vi "Print Console.vi"() -> ()   [LabVIEW 2016]
doc: "This print queue console simulates the control of print job submissions and monitors the status of the print jobs being processed."
uses:
  Print Indicators.ctl
  Print Processing States.ctl
  <vilib>/Utility/error.llb/DialogType.ctl
panel:
  out "Print Indicators":T1={"Waiting"=TRUE, "Initializing"=FALSE, "Printing"=FALSE, "Job Number"=0}
  out "Queued Print Jobs":i32(slide) scale=0.0..25.0
  in  "Queue Event":bool
  in  "Stop":bool
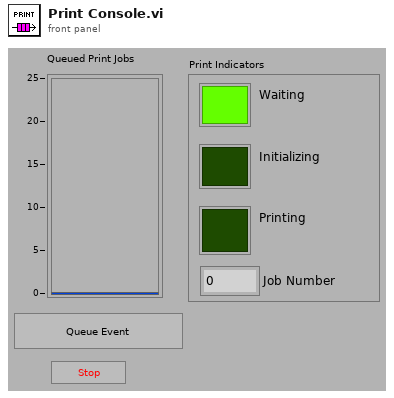
[diagram p1: front panel]
types:
  T1 = typedef "Print Indicators.ctl" = cluster{"Waiting":bool, "Initializing":bool, "Printing":bool, "Job Number":i32}
  T2 = typedef "DialogType.ctl" = u16
  T3 = typedef "Print Processing States.ctl" = enum16{"Wait", "Initialize Setup", "Setup", "Initialize Print", "Print", "Shutdown"}
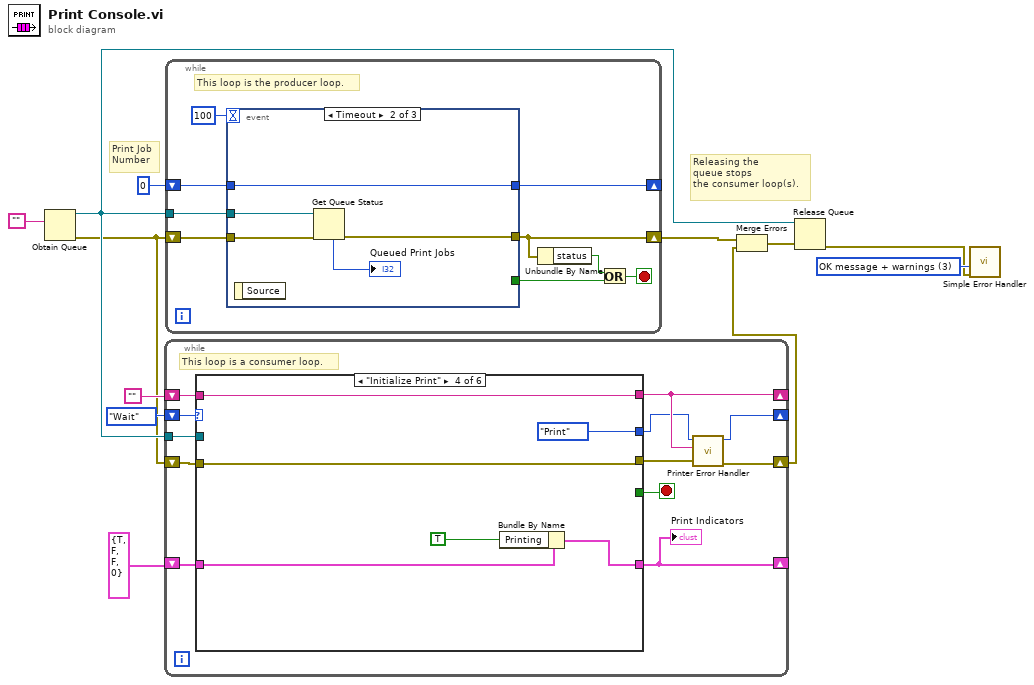
[diagram p0: block diagram]
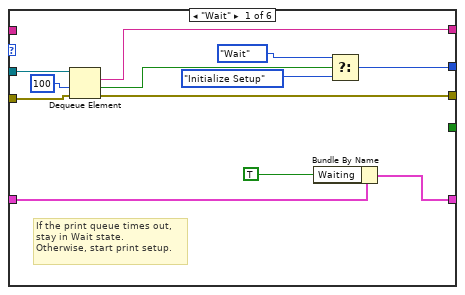
[diagram p2: hidden frame]
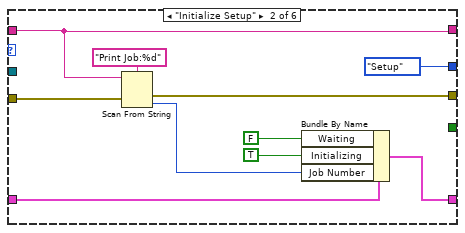
[diagram p3: hidden frame]
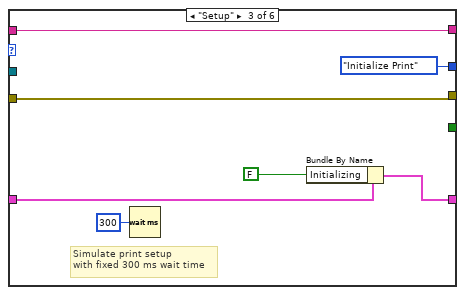
[diagram p4: hidden frame]
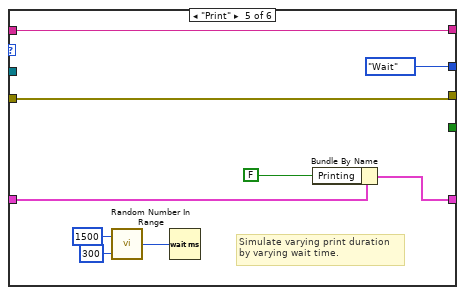
[diagram p5: hidden frame]
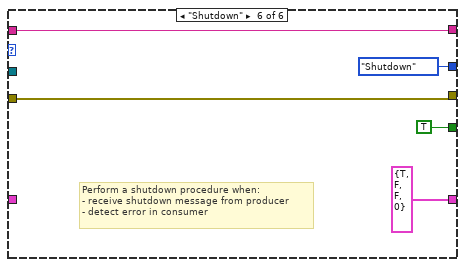
[diagram p6: hidden frame]
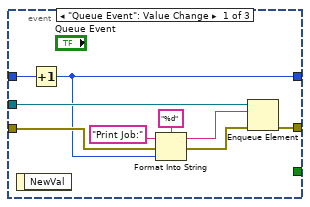
[diagram p7: hidden frame]
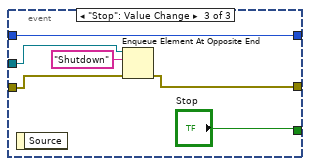
[diagram p8: hidden frame]
diagram:
  w5 = T2 3 items=["no dialog", "OK message", "continue or stop message", "OK message + warnings", "continue/stop + warnings"] ("type of dialog (OK msg:1)")
  # "Print Job\nNumber"
  # "Releasing the\nqueue stops\nthe consumer loop(s)."
  n1 = Obtain Queue(element data type="") -> (queue out=w11:refnum<queue>, error out=w6:errorcluster)  [unwired: 4 in, 1 out]
  n2 = while {
    tunnel: w11 -> [w24]
    shift-right: [w13] -> _
    shift-left: Print_Processing_States."Wait" ("Enum") -> [w23]
    shift-right: [w21] -> _
    shift-left: T1 {"Waiting"=TRUE, "Initializing"=FALSE, "Printing"=FALSE, "Job Number"=0} ("Print LEDs") -> [w22]
    shift-right: [w15] -> _
    shift-left: "" -> [w20]
    shift-right: [w16] -> w1
    shift-left: w6 -> [w19]
    stop <- w18 stop-if-true
    # "This loop is a consumer loop."
    n3 = case shown="\"Initialize Print\"" w23 {
      tunnel: w24 -> [w36 _ _ _ _ _]
      tunnel: [w35 w38 w47 w54 w60 w70] -> w17
      tunnel: w22 -> [w30 w45 w52 w58 w67 _]
      tunnel: [w29 w44 w51 w57 w66 T1 {"Waiting"=TRUE, "Initializing"=FALSE, "Printing"=FALSE, "Job Number"=0} ("Print LEDs")] -> w21
      tunnel: [w27 Print_Processing_States."Setup" ("Enum") Print_Processing_States."Initialize Print" ("Enum") Print_Processing_States."Print" ("Enum") Print_Processing_States."Wait" ("Enum") Print_Processing_States."Shutdown" ("Enum")] -> w14
      tunnel: [w26 w41 w48 w55 w61 w71] -> w15
      tunnel: w20 -> [_ w41 w48 w55 w61 w71]
      tunnel: w19 -> [w25 w37 w47 w54 w60 w70]
      tunnel: [_ _ _ _ _ TRUE] -> w18
      frame "Wait" {
        # "If the print queue times out, \nstay in Wait state.\nOtherwise, start print setup."
        n4 = Dequeue Element(queue=w36, timeout in ms (-1)=100, error in (no error)=w25) -> (element=w26:string, timed out?=w28:bool, error out=w35:errorcluster)  [unwired: 1 out]
        n5 = Bundle By Name(cluster=w30, "Waiting"=TRUE ("Waiting for\nnew job...")) -> (w29:T1)
        n6 = Select(t=Print_Processing_States."Wait" ("Enum"), s=w28, f=Print_Processing_States."Initialize Setup" ("Enum")) -> (s? t:f=w27:T3)
      }
      frame "Initialize Setup" {
        n7 = Scan From String(format string="Print Job:%d", input string=w41, error in=w37) -> (error out=w38:errorcluster, output 1=w39:i32)  [unwired: 2 in, 2 out]
        n8 = Bundle By Name(cluster=w45, "Waiting"=FALSE ("Waiting for\nnew job..."), "Initializing"=TRUE ("Waiting for\nnew job..."), "Job Number"=w39) -> (w44:T1)
      }
      frame "Setup" {
        # "Simulate print setup\nwith fixed 300 ms wait time"
        n9 = Wait (ms)(milliseconds to wait=u32 300) -> ()  [unwired: 1 out]
        n10 = Bundle By Name(cluster=w52, "Initializing"=FALSE ("Waiting for\nnew job...")) -> (w51:T1)
      }
      frame "Initialize Print" {
        n11 = Bundle By Name(cluster=w58, "Printing"=TRUE ("Waiting for\nnew job...")) -> (w57:T1)
      }
      frame "Print" {
        # "Simulate varying print duration\nby varying wait time."
        n12 = call "Random Number In Range.vi"("Lower Limit"=u32 300, "Upper Limit"=u32 1500) -> ("Random #"=w62:u32)
        n13 = Wait (ms)(milliseconds to wait=w62) -> ()  [unwired: 1 out]
        n14 = Bundle By Name(cluster=w67, "Printing"=FALSE ("Waiting for\nnew job...")) -> (w66:T1)
      }
      frame "Shutdown" {
        # "Perform a shutdown procedure when:\n- receive shutdown message from producer\n- detect error in consumer"
      }
    }
    "Print Indicators" <- w21
    n15 = call "Printer Error Handler.vi"("error in (no error)"=w17, "Queue Data"=w15, "State In"=w14) -> ("error out"=w16:errorcluster, "Next State"=w13:T3)  [unwired: 7 in]
  }
  n16 = while {
    tunnel: w11 -> [w82]
    shift-right: [w76] -> _
    shift-left: 0 -> [w77]
    shift-right: [w75] -> w4
    shift-left: w6 -> [w74]
    stop <- w80 stop-if-true
    # "This loop is the producer loop."
    n17 = event shown="[1] Timeout" {
      selector: _ -> [_ _ _]
      dyn-events: _ -> [_ _ _]
      timeout: 100 -> [_ _ _]
      tunnel: w82 -> [w91 w94 w97]
      tunnel: w74 -> [w89 w95 w100]
      tunnel: [w90 w93 w99] -> w75
      tunnel: [_ _ "Stop"] -> w81
      tunnel: w77 -> [w85 w92 w101]
      tunnel: [w83 w92 w101] -> w76
      event "Queue Event": Value Change {
        n18 = event-data() -> ()  [unwired: 1 in, 1 out]
        n19 = Increment(x=w85) -> (x+1=w83:i32)
        n20 = Format Into String(format string="%d", initial string="Print Job:", error in=w89, w83) -> (resulting string=w84:string, error out=w88:errorcluster)
        n21 = Enqueue Element(queue=w91, element=w84, error in (no error)=w88) -> (error out=w90:errorcluster)  [unwired: 1 in, 2 out]
      }
      event Timeout {
        n22 = event-data() -> ()  [unwired: 1 in, 1 out]
        n23 = Get Queue Status(queue=w94, error in (no error)=w95) -> (error out=w93:errorcluster, # elements in queue=→"Queued Print Jobs":i32)  [unwired: 1 in, 6 out]
      }
      event "Stop": Value Change {
        n24 = event-data() -> ()  [unwired: 1 in, 1 out]
        n25 = Enqueue Element At Opposite End(queue=w97, element="Shutdown", error in (no error)=w100) -> (error out=w99:errorcluster)  [unwired: 1 in, 2 out]
      }
    }
    n26 = Unbundle By Name(w75) -> ("status"=w79:bool)
    n27 = Or(x=w79, y=w81) -> (x .or. y?=w80:bool)
  }
  n28 = Merge Errors(w4, w1) -> (w3:errorcluster)
  n29 = Release Queue(queue=w11, error in (no error)=w3) -> (error out=w2:errorcluster)  [unwired: 1 in, 2 out]
  n30 = call <vilib>:"Simple Error Handler.vi"("type of dialog (OK msg:1)"=w5, "error in (no error)"=w2) -> ()  [unwired: 3 in, 5 out]
